vi "CreateFrames.vi"(8 "error in (no error)":errorcluster, 11 "DAQList in":refnum<class "DAQList.lvclass">) -> (0 "error out":errorcluster, 3 "DAQList out":refnum<class "DAQList.lvclass">)   [LabVIEW 2019, in "XCP_DaqDtoId.lvlib" / "DAQList.lvclass"]
uses:
  DAQList.lvclass
  DAQList.lvclass/DAQList.ctl
  <vilib>/Utility/error.llb/Error Cluster From Error Code.vi
  <vilib>/xnet/xnet.llb/XNET Database Create (Frame).vi
  <vilib>/ErrorRing/Error Ring.xnode
  <resource>/objmgr/xnet.rc
panel:
  out "Array":refnum<k21>[](array[refnum])
  in  "Save?":bool
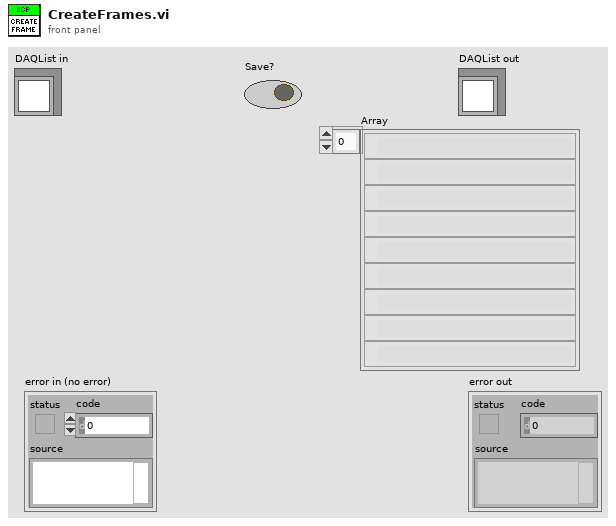
[diagram p1: front panel]
types:
  T1 = cluster{"Frame name":string, "Identifier":u32, "Payload Length":u32, "Timing Type":u32, "Transmit Time":dbl, "Extended Identifier?":bool, "Comment":string}[]
  T2 = cluster{"Frame name":string, "Identifier":u32, "Payload Length":i32, "Timing Type":u32, "Transmit Time":dbl, "Extended Identifier?":bool, "Comment":string}
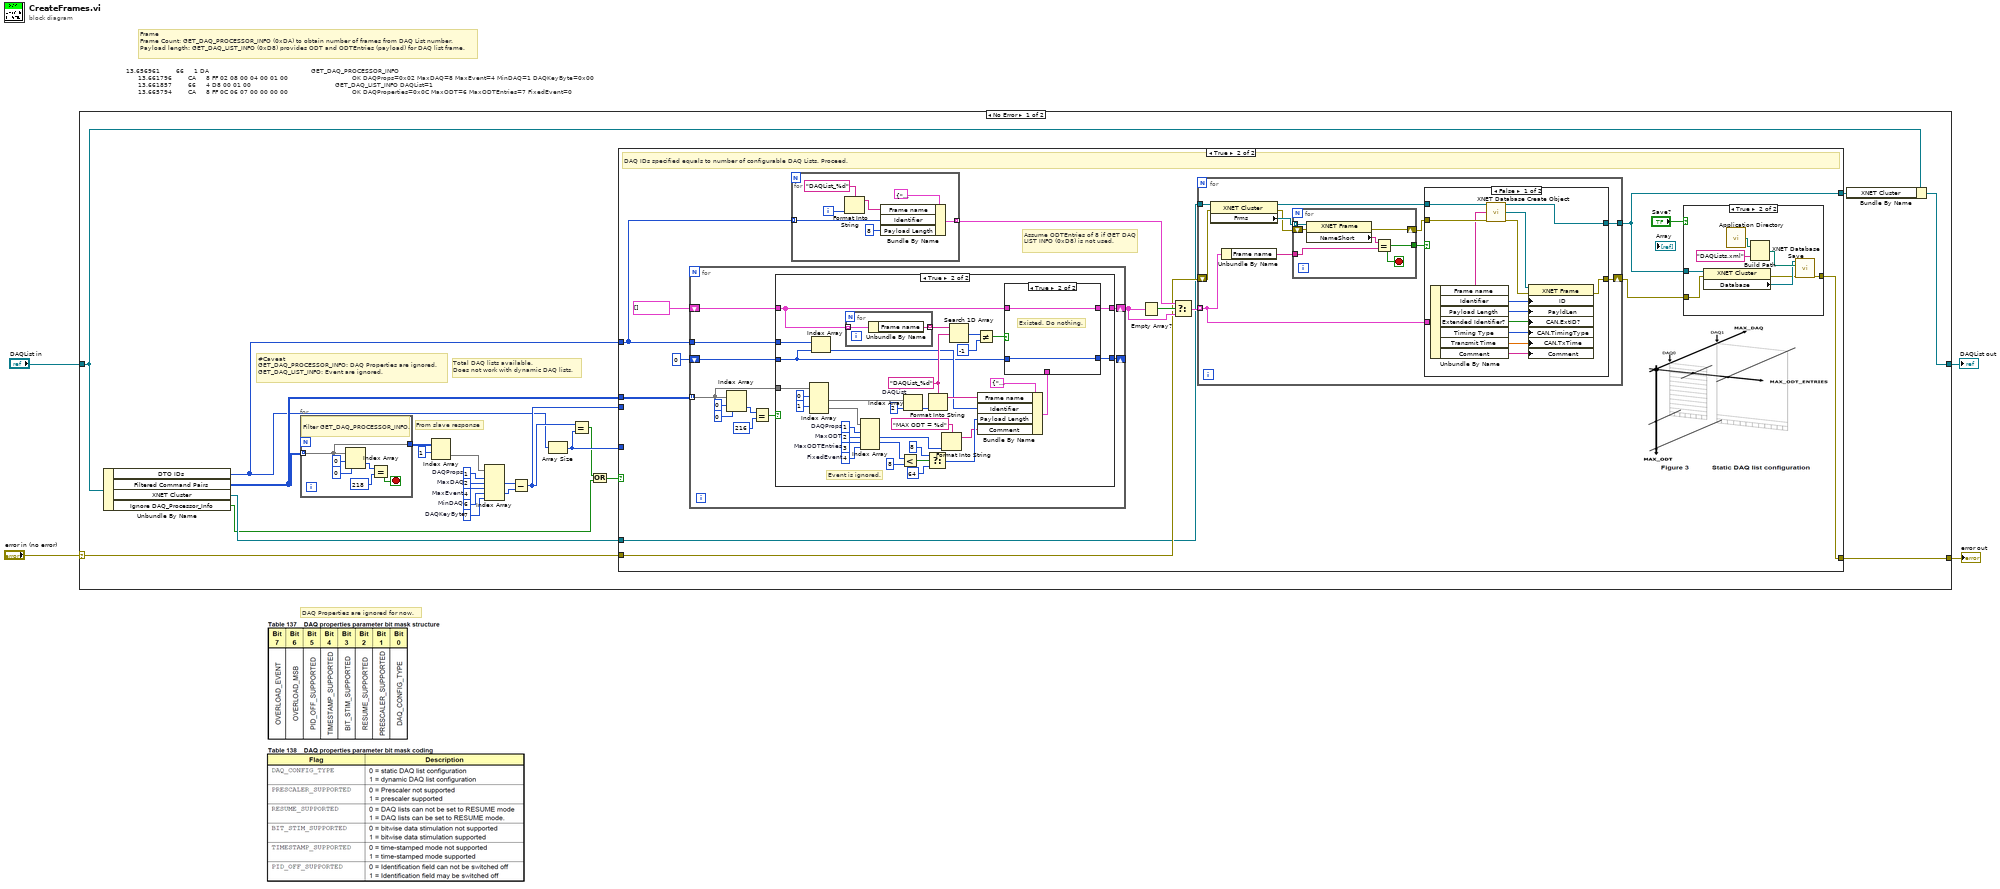
[diagram p0: block diagram]
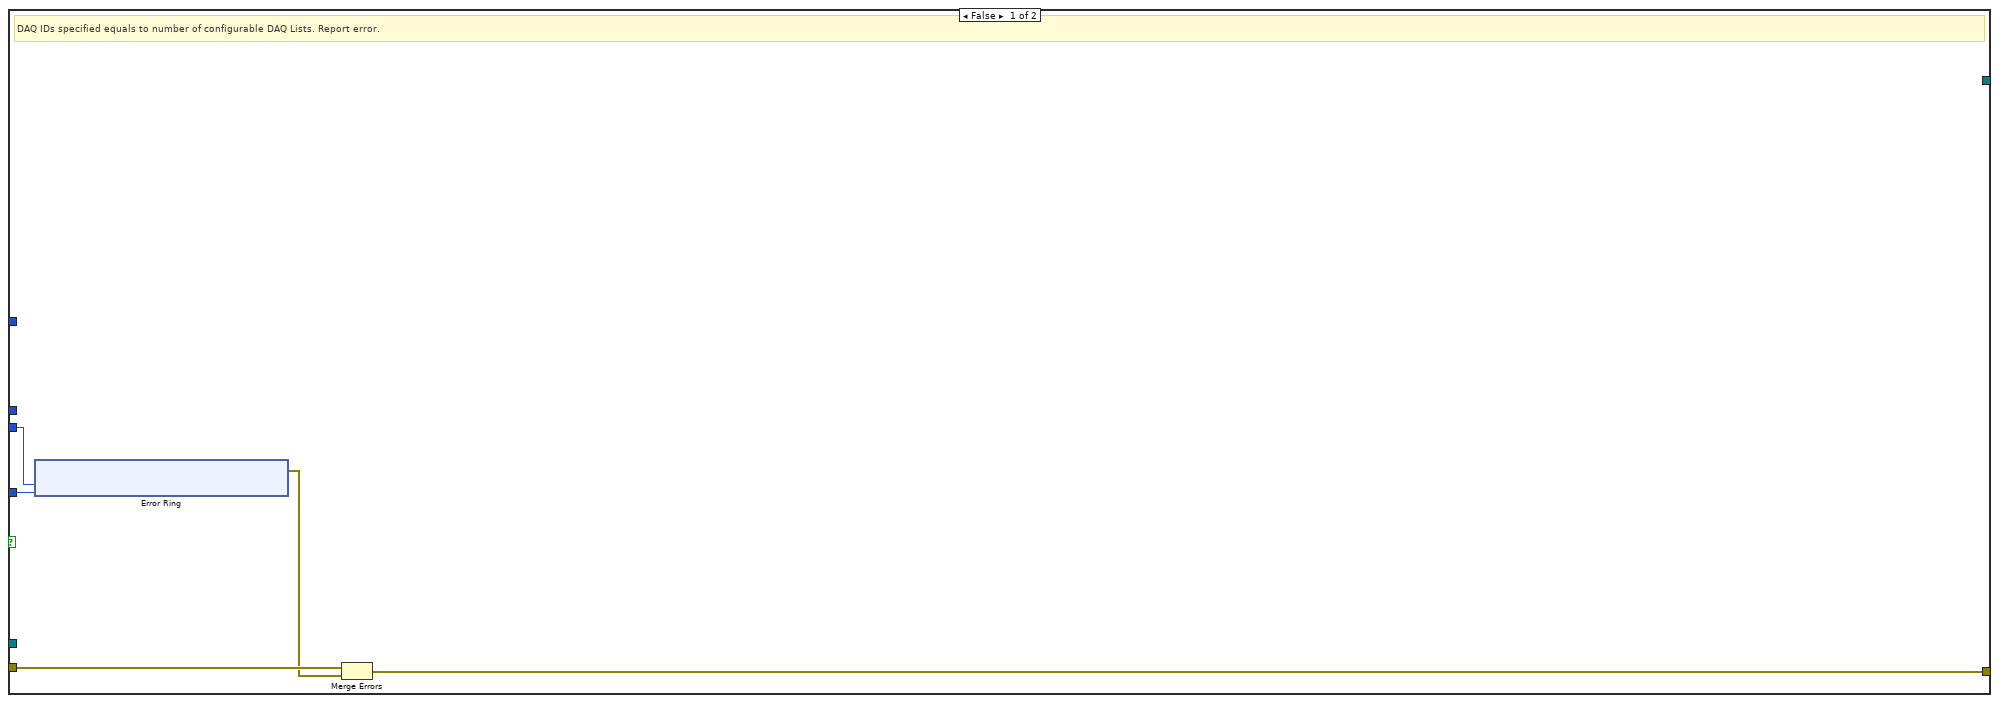
[diagram p2: hidden frame]
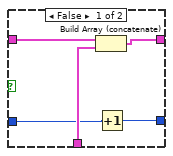
[diagram p4: hidden frame]
diagram:
  # "13.656961        66     1 DA                                                   GET_DAQ_PROCESSOR_INFO\n      13.661796        CA     8 FF 02 08 00 04 00 01 00                                OK DAQProps=0x02 MaxDAQ=8 MaxEvent=4 MinDAQ=1 DAQKeyByte=0x00\n      13.661857        66     4 D8 00 01 00                                          GET_DAQ_LIST_INFO DAQList=1\n      13.665794        CA     8 FF 0C 06 07 00 00 00 00                                OK DAQProperties=0x0C MaxODT=6 MaxODTEntries=7 FixedEvent=0"
  # "Frame\nFrame Count: GET_DAQ_PROCESSOR_INFO (0xDA) to obtain number of frames from DAQ List number.\nPayload length: GET_DAQ_LIST_INFO (0xD8) provides ODT and ODTEntries (payload) for DAQ list frame."
  # "DAQ Properties are ignored for now."
  n1 = case shown="No Error" "error in (no error)" {
    selector: "error in (no error)" -> [w11 w167]
    tunnel: [w15 w167] -> w3
    tunnel: [w10 w166] -> w1
    tunnel: "DAQList in" -> [w9 w166]
    frame No Error {
      w20 = 7  # DAQKeyByte
      w21 = 6  # MinDAQ
      w22 = 4  # MaxEvent
      w23 = 2  # MaxDAQ
      w24 = 1  # DAQProps
      # "#Caveat\nGET_DAQ_PROCESSOR_INFO: DAQ Properties are ignored.\nGET_DAQ_LIST_INFO: Event are ignored."
      # "Total DAQ lists available.\nDoes not work with dynamic DAQ lists."
      # "From slave response"
      n2 = Unbundle By Name(w9) -> ("DTO IDs"=w13:u32[], "Filtered Command Pairs"=w14:u8[][][], "XNET Cluster"=w12:refnum<k21>, "Ignore DAQ_Processor_Info"=w6:bool)
      n3 = for {
        tunnel: w14 -> [w29] mode=indexing
        tunnel: [w29] -> w27
        stop <- w28 stop-if-true
        # "Filter GET_DAQ_PROCESSOR_INFO."
        n4 = Index Array(array=w29, index (row)=0, index (col)=0 ("disabled index (col)")) -> (element=w31:u8)
        n5 = Equal?(x=w31, y=u8 218 ("element")) -> (x = y?=w28:bool)
      }
      n6 = Index Array(array=w27, index (row)=1) -> (element=w25:u8[])  [unwired: 1 in]
      n7 = Index Array(array=w25, index #1=w24, index #2=w23, index #3=w22, index #4=w21, index #5=w20) -> (element #2=w19:u8, element #4=w18:u8)  [unwired: 3 out]
      n8 = Subtract(x=w19, y=w18) -> (x-y=w17:u8)
      n9 = Array Size(array=w13) -> (size(s)=w16:i32)
      n10 = Equal?(x=w17, y=w16) -> (x = y?=w7:bool)
      n11 = Or(x=w7, y=w6) -> (x .or. y?=w5:bool)
      n12 = case shown="True" w5 {
        tunnel: w14 -> [_ w60]
        tunnel: w13 -> [_ w50]
        tunnel: [w35 w56] -> w15
        tunnel: w11 -> [w37 w51]
        tunnel: w17 -> [w38 _]
        tunnel: w16 -> [w34 _]
        tunnel: w12 -> [_ w48]
        tunnel: [_ w47] -> w8
        frame False {
          # "DAQ IDs specified equals to number of configurable DAQ Lists. Report error."
          n13 = xnode "Error Ring"("parameter 0"=w38, "parameter 1"=w34) -> ("error out"=w36:errorcluster)
          n14 = Merge Errors(w37, w36) -> (w35:errorcluster)
        }
        frame True {
          # "Assume ODTEntries of 8 if GET DAQ LIST INFO (0xD8) is not used."
          # "DAQ IDs specified equals to number of configurable DAQ Lists. Proceed."
          n15 = for {
            tunnel: w60 -> [w78] mode=indexing
            shift-right: [w70] -> w53
            shift-left: T1 [] -> [w71]
            shift-right: [w68] -> _
            shift-left: 0 ("y") -> [w69]
            tunnel: w50 -> [w72]
            n16 = Index Array(array=w78, index (row)=0, index (col)=0 ("disabled index (col)")) -> (element=w75:u8)
            n17 = Equal?(x=w75, y=u8 216 ("element")) -> (x = y?=w73:bool)
            n18 = case shown="True" w73 {
              tunnel: w78 -> [_ w108]
              tunnel: w72 -> [_ w87]
              tunnel: w71 -> [w80 w90]
              tunnel: [w80 w88] -> w70
              tunnel: w69 -> [w79 w84]
              tunnel: [w79 w85] -> w68
              frame False {
              }
              frame True {
                w93 = "DAQList_%d"
                w105 = 2  # DAQList
                w114 = 4  # FixedEvent
                w113 = 3  # MaxODTEntries
                w112 = 2  # MaxODT
                w111 = 1  # DAQProps
                # "Event is ignored."
                n19 = Index Array(array=w108, index (row) #1=0 ("index (row)"), index (row) #2=1 ("index (row)")) -> (element #1=w106:u8[], element #2=w110:u8[])  [unwired: 2 in]
                n20 = Index Array(array=w87, index=w84) -> (element=w86:u32)
                n21 = for {
                  tunnel: w90 -> [w123] mode=indexing
                  tunnel: [w122] -> w94 mode=indexing
                  n22 = Unbundle By Name(w123) -> ("Frame name"=w122:string)
                }
                n23 = Index Array(array=w110, index #1=w111, index #2=w112, index #3=w113, index #4=w114) -> (element #2=w82:u8, element #3=w101:u8)  [unwired: 2 out]
                n24 = Less?(x=w101, y=u8 8) -> (x < y?=w99:bool)
                n25 = Index Array(array=w106, index=w105) -> (element=w104:u8)
                n26 = Select(t=8 ("y"), s=w99, f=64) -> (s? t:f=w98:i32)
                n27 = Format Into String(format string=w93, w104) -> (resulting string=w102:string)  [unwired: 2 in, 1 out]
                n28 = Format Into String(format string="MAX ODT = %d", w82) -> (resulting string=w81:string)  [unwired: 2 in, 1 out]
                n29 = Search 1D Array(1D array=w94, element=w93) -> (index of element=w92:i32)  [unwired: 1 in]
                n30 = Not Equal?(x=w92, y=-1) -> (x != y?=w89:bool)
                n31 = Bundle By Name(cluster=T2 {"Frame name"="", "Identifier"=0, "Payload Length"=0, "Timing Type"=1, "Transmit Time"=0.001, "Extended Identifier?"=FALSE, "Comment"=""} ("CAN Frame"), "Frame name"=w102, "Identifier"=w86, "Payload Length"=w98, "Comment"=w81) -> (w95:T2)
                n32 = case shown="True" w89 {
                  tunnel: w95 -> [w119 _]
                  tunnel: w90 -> [w118 w121]
                  tunnel: [w117 w121] -> w88
                  tunnel: [w116 w120] -> w85
                  tunnel: w84 -> [w115 w120]
                  frame False {
                    n33 = Build Array (concatenate)(w118, w119) -> (w117:T1)
                    n34 = Increment(x=w115) -> (x+1=w116:i32)
                  }
                  frame True {
                    # "Existed. Do nothing."
                  }
                }
              }
            }
          }
          n35 = for {
            tunnel: w50 -> [w63] mode=indexing
            tunnel: [w61] -> w52 mode=indexing
            i -> [w65]
            n36 = Format Into String(format string="DAQList_%d", w65) -> (resulting string=w64:string)  [unwired: 2 in, 1 out]
            n37 = Bundle By Name(cluster=T2 {"Frame name"="", "Identifier"=0, "Payload Length"=0, "Timing Type"=1, "Transmit Time"=0.01, "Extended Identifier?"=FALSE, "Comment"=""} ("CAN Frame"), "Frame name"=w64, "Identifier"=w63, "Payload Length"=8 ("y")) -> (w61:T2)
          }
          n38 = Empty Array?(array=w53) -> (empty?=w55:bool)
          n39 = Select(t=w52, s=w55, f=w53) -> (s? t:f=w54:T1)
          n40 = for {
            tunnel: w48 -> [w132]
            shift-right: [w133] -> w57
            shift-left: w51 -> [w131]
            tunnel: w54 -> [w127] mode=indexing
            tunnel: [w134] -> w47
            n41 = property class="XNET Cluster"(reference=w132, error in=w131) -> (reference out=w130:refnum<k21>, error out=w125:errorcluster, "Frms"=w129:refnum<k21>[])
            n42 = Unbundle By Name(w127) -> ("Frame name"=w126:string)
            n43 = for {
              tunnel: w129 -> [w155] mode=indexing
              tunnel: w126 -> [w154]
              shift-right: [w156] -> w128
              shift-left: w125 -> [w152]
              tunnel: [w151] -> w124
              stop <- w151 stop-if-true
              n44 = property class="XNET Frame"(reference=w155, error in=w152) -> (error out=w156:errorcluster, "NameShort"=w153:string)  [unwired: 1 out]
              n45 = Equal?(x=w153, y=w154) -> (x = y?=w151:bool)
            }
            n46 = case shown="False" w124 {
              tunnel: [w141 w150] -> w134
              tunnel: [w139 w149] -> w133
              tunnel: w130 -> [w138 w150]
              tunnel: w128 -> [w137 w149]
              tunnel: w127 -> [w136 _]
              frame False {
                n47 = Unbundle By Name(w136) -> ("Frame name"=w135:string, "Identifier"=w146:u32, "Payload Length"=w145:u32, "Extended Identifier?"=w144:bool, "Timing Type"=w143:u32, "Transmit Time"=w142:dbl, "Comment"=w148:string)
                n48 = call-poly <vilib>:"XNET Database Create Object.vi"("cluster in"=w138, "frame name"=w135, "error in (no error)"=w137) -> ("cluster out"=w141:refnum<k21>, "frame out"=w140:refnum<k21>, "error out"=w147:errorcluster)  [unwired: 10 in]
                n49 = property class="XNET Frame"(reference=w140, error in=w147, "ID"=w146, "PayldLen"=w145, "CAN.ExtID?"=w144, "CAN.TimingType"=w143, "CAN.TxTime"=w142, "Comment"=w148) -> (error out=w139:errorcluster)  [unwired: 1 out]
              }
              frame True {
                # "DAQ List already added. Do nothing."
              }
            }
          }
          n50 = case shown="True" "Save?" {
            tunnel: w47 -> [_ w165]
            tunnel: w57 -> [w157 w164]
            tunnel: [w157 w163] -> w56
            frame False {
            }
            frame True {
              n51 = property class="XNET Cluster"(reference=w165, error in=w164) -> (error out=w158:errorcluster, "Database"=w159:refnum<k21>)  [unwired: 1 out]
              n52 = call <vilib>:"Application Directory.vi"() -> ("Application Directory"=w161:path)
              n53 = Build Path(base path=w161, name or relative path="DAQLists.xml") -> (appended path=w160:path)
              n54 = call <vilib>:"XNET Database Save.vi"("database in"=w159, "filepath (empty)"=w160, "error in (no error)"=w158) -> ("error out"=w163:errorcluster)  [unwired: 11 in, 1 out]
            }
          }
        }
      }
      n55 = Bundle By Name(cluster=w9, "XNET Cluster"=w8) -> (w10:refnum<class "DAQList.lvclass">)
    }
    frame Error {
    }
  }
  "error out" <- w3
  "DAQList out" <- w1
